vi "Get Connection Info.vi"(8 "error in (no error)":errorcluster, 11 "UDL Connection in":refnum<class "UDL Connection.lvclass">) -> (0 "error out":errorcluster, 1 "User":string, 2 "*.uld file path":path, 3 "UDL Connection out":refnum<class "UDL Connection.lvclass">, 4 "Password":string)   [LabVIEW 2020, in "ADODB.lvlib" / "UDL Connection.lvclass"]
uses:
  UDL Connection.lvclass
  UDL Connection.lvclass/UDL Connection.ctl
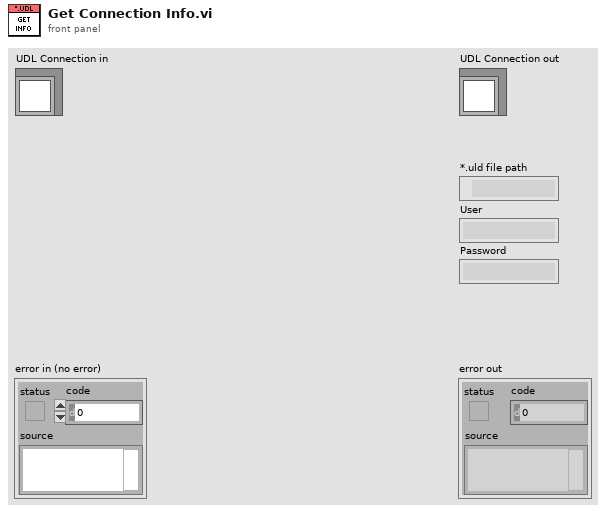
[diagram p1: front panel]
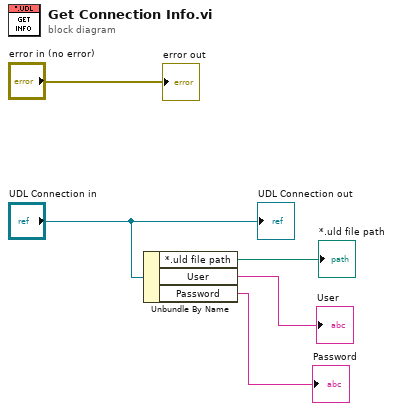
[diagram p0: block diagram]
diagram:
  n1 = Unbundle By Name("UDL Connection in") -> ("*.uld file path"=→"*.uld file path":path, "User"=→"User":string, "Password"=→"Password":string)
  "error out" <- "error in (no error)"
  "UDL Connection out" <- "UDL Connection in"
